vi "Connect.vi"(8 "error in (no error)":errorcluster, 11 "OXY_SCPI Resource In":string="192.168.0.10") -> (0 "error out":errorcluster, 3 "OXY_SCPI Resource Out":refnum<visa-resource-name>)   [LabVIEW 2020, in "OXYGEN_Datastream.lvlib"]
uses:
  OXYGEN_Datastream.lvlib
  Application Control/SubVIs/CommunicationFormat_SetActivationOutputHeader.vi
  Application Control/SubVIs/CommunicationFormat_SetHeaderLength.vi
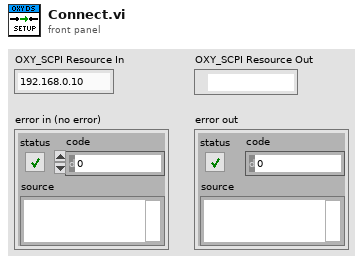
[diagram p1: front panel]
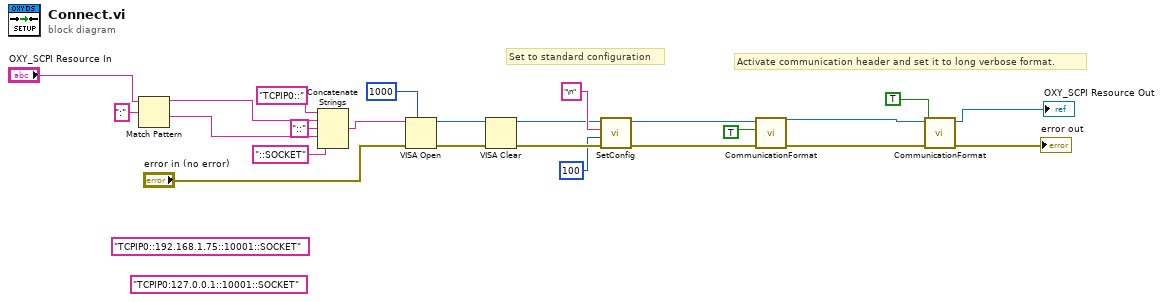
[diagram p0: block diagram]
diagram:
  (unwired) "TCPIP0:127.0.0.1::10001::SOCKET" ("string")
  (unwired) "TCPIP0::192.168.1.75::10001::SOCKET" ("string")
  # "Activate communication header and set it to long verbose format."
  # "Set to standard configuration"
  n1 = Match Pattern(string="OXY_SCPI Resource In", regular expression=":") -> (before substring=w18:string, after substring=w17:string)  [unwired: 1 in, 2 out]
  n2 = Concatenate Strings("TCPIP0::" ("string"), w18, "::" ("string"), w17, "::SOCKET" ("string")) -> (w14:string)
  n3 = VISA Open(timeout (0)=u32 1000 ("VISA Open timeout (0)"), error in (no error)="error in (no error)", VISA resource name=w14) -> (VISA resource name=w12:refnum<visa-resource-name>, error out=w13:errorcluster)  [unwired: 2 in]
  n4 = VISA Clear(VISA resource name=w12, error in (no error)=w13) -> (VISA resource name out=w11:refnum<visa-resource-name>, error out=w10:errorcluster)
  n5 = call "SetConfig.vi"("error in (no error)"=w10, "Timeout"=u32 100, "TermChr"="\n", "OXY_SCPI Reseource In"=w11) -> ("error out"=w7:errorcluster, "OXY_SCPI Reseource Out"=w6:refnum<visa-resource-name>)  [unwired: 6 in]
  n6 = call-poly "CommunicationFormat.vi"("error in (no error)"=w7, "Activate Header"=TRUE, "OXYGEN Ref In"=w6) -> ("error out"=w1:errorcluster, "OXYGEN Ref Out"=w4:refnum<visa-resource-name>)  [unwired: 6 in, 1 out]
  n7 = call-poly "CommunicationFormat.vi"("error in (no error)"=w1, "Long Communication Header?"=TRUE, "OXYGEN Ref In"=w4) -> ("error out"=→"error out":errorcluster, "OXYGEN Ref Out"=→"OXY_SCPI Resource Out":refnum<visa-resource-name>)  [unwired: 6 in, 1 out]
